vi "xijk_create_graphs_emission.vi"(7 "plot settings in":cluster{"axes in":T1, "plot colors in":T2} {"axes in"."precision of results" max=8 step=1}, 8 "error in":errorcluster, 11 "spectra in":T3) -> (0 "error out":errorcluster, 1 "Filter cube 2 emission":cluster{"Y":dbl[], "Y":dbl[]}[](graph), 3 "Filter cube 1 emission":cluster{"Y":dbl[], "Y":dbl[]}[](graph))   [LabVIEW 2010]
uses:
  Type Def/spectrum_table_control.ctl
  Type Def/axis_parameters.ctl
  revised version/Type Def/color_parameters.ctl
panel:
  # "Dichroic"
  # "Ex/Em filter"
  # "Fluorophore 1"
  # "Fluorophore 2"
  # "Laser /\nextra Em filter"
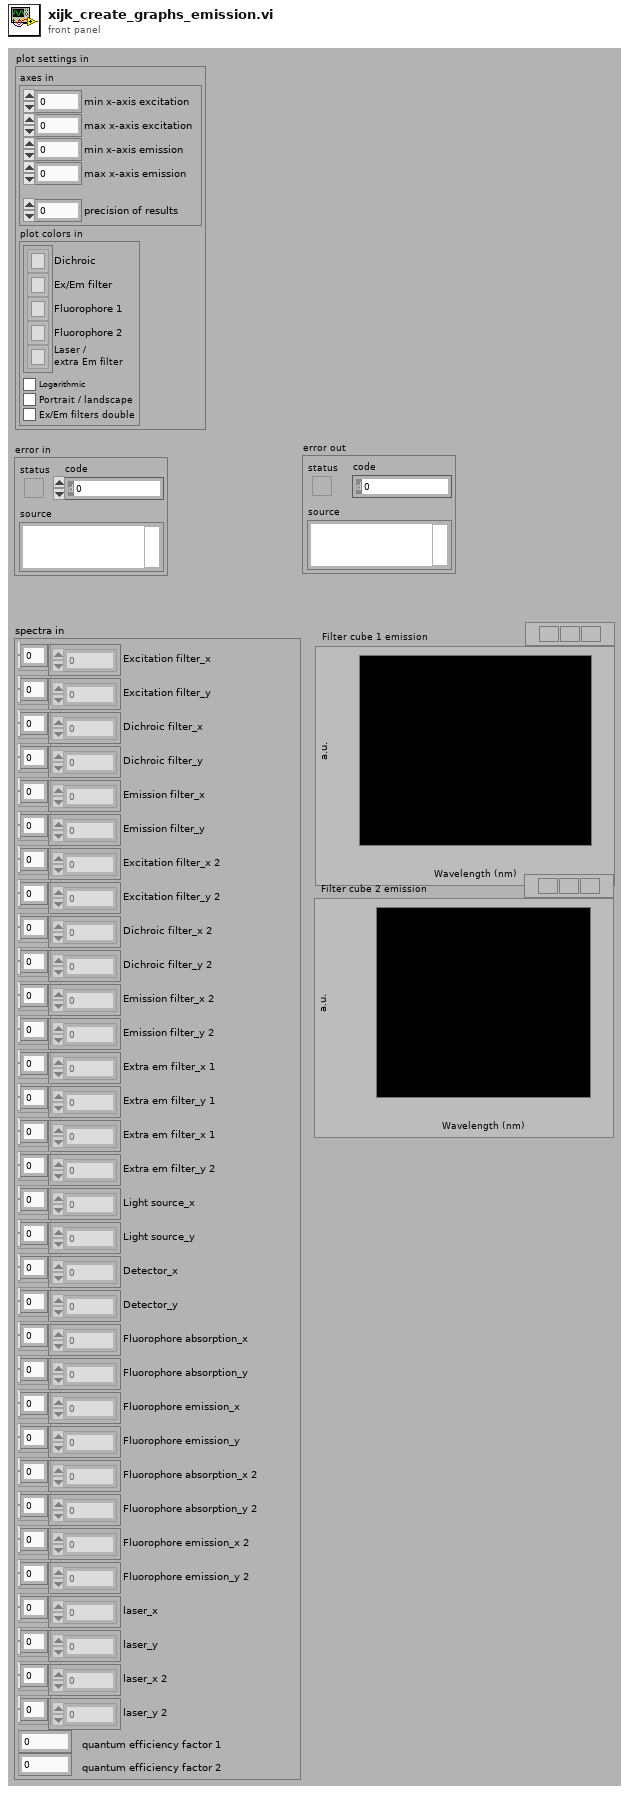
[diagram p1: front panel]
types:
  T1 = typedef "axis_parameters.ctl" = cluster{"min x-axis excitation":u16, "max x-axis excitation":u16, "min x-axis emission":u16, "max x-axis emission":u16, "precision of results":u8}
  T2 = typedef "color_parameters.ctl" = cluster{"Line colors":u32[], "Lanscape Portrait":bool, "Plot logarithmic":bool, "Ex/Em filters double":bool}
  T3 = typedef "spectrum_table_control.ctl" = cluster{"Excitation filter_x":i16[], "Excitation filter_y":dbl[], "Dichroic filter_x":i16[], "Dichroic filter_y":dbl[], "Emission filter_x":i16[], "Emission filter_y":dbl[], "Excitation filter_x 2":i16[], "Excitation filter_y 2":dbl[], "Dichroic filter_x 2":i16[], "Dichroic filter_y 2":dbl[], "Emission filter_x 2":i16[], "Emission filter_y 2":dbl[], "Extra em filter_x 1":i16[], "Extra em filter_y 1":dbl[], "Extra em filter_x 1":i16[], "Extra em filter_y 2":dbl[], "Light source_x":i16[], "Light source_y":dbl[], "Detector_x":i16[], "Detector_y":dbl[], "Fluorophore absorption_x":i16[], "Fluorophore absorption_y":dbl[], "Fluorophore emission_x":i16[], "Fluorophore emission_y":dbl[], "Fluorophore absorption_x 2":i16[], "Fluorophore absorption_y 2":dbl[], "Fluorophore emission_x 2":i16[], "Fluorophore emission_y 2":dbl[], "laser_x":i16[], "laser_y":dbl[], "laser_x 2":i16[], "laser_y 2":dbl[], "quantum efficiency factor 1":dbl, "quantum efficiency factor 2":dbl}
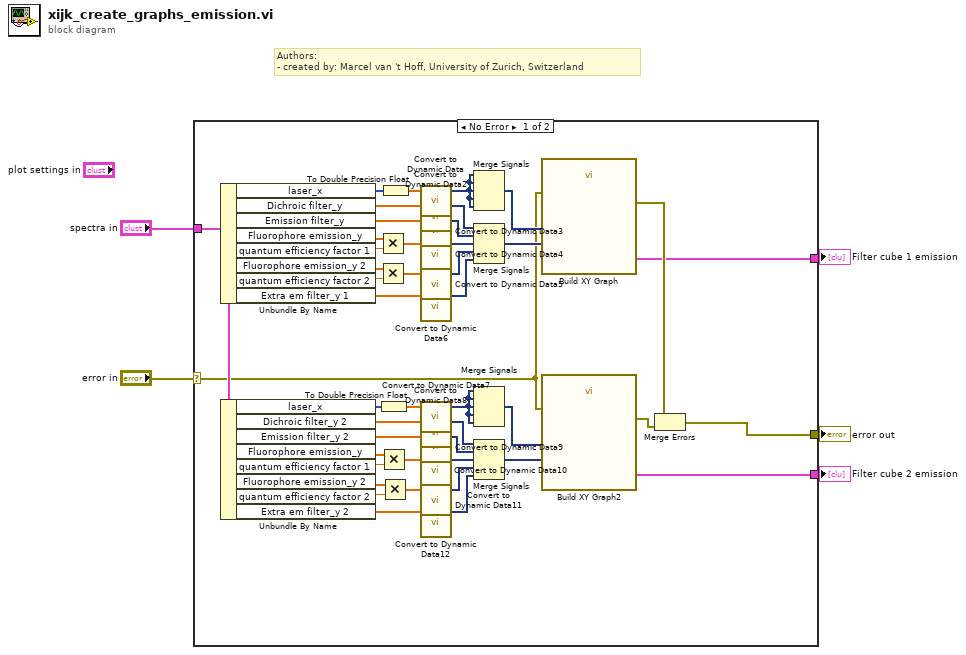
[diagram p0: block diagram]
diagram:
  # "Authors: \n- created by: Marcel van 't Hoff, University of Zurich, Switzerland"
  n1 = case shown="No Error" "error in" {
    selector: "error in" -> [w22 w51]
    tunnel: "spectra in" -> [w50 _]
    tunnel: [w23 w51] -> w4
    tunnel: [w6 _] -> w2
    tunnel: [w21 _] -> w1
    frame No Error {
      n2 = Unbundle By Name(w50) -> ("laser_x"=w49:i16[], "Dichroic filter_y"=w48:dbl[], "Emission filter_y"=w45:dbl[], "Fluorophore emission_y"=w43:dbl[], "quantum efficiency factor 1"=w16:dbl, "Fluorophore emission_y 2"=w18:dbl[], "quantum efficiency factor 2"=w14:dbl, "Extra em filter_y 1"=w40:dbl[])
      n3 = Unbundle By Name(w50) -> ("laser_x"=w29:i16[], "Dichroic filter_y 2"=w28:dbl[], "Emission filter_y 2"=w27:dbl[], "Fluorophore emission_y"=w8:dbl[], "quantum efficiency factor 1"=w12:dbl, "Fluorophore emission_y 2"=w10:dbl[], "quantum efficiency factor 2"=w11:dbl, "Extra em filter_y 2"=w26:dbl[])
      n4 = Multiply(x=w43, y=w16) -> (x*y=w17:dbl[])
      n5 = Multiply(x=w18, y=w14) -> (x*y=w15:dbl[])
      n6 = To Double Precision Float(number=w29) -> (double precision float=w20:dbl[])
      n7 = Multiply(x=w8, y=w12) -> (x*y=w7:dbl[])
      n8 = Multiply(x=w10, y=w11) -> (x*y=w9:dbl[])
      n9 = To Double Precision Float(number=w49) -> (double precision float=w19:dbl[])
      n10 = call "Convert to Dynamic Data"("Array"=w19) -> ("Dynamic Data Type"=w38:dynamicdata)  [unwired: 3 in]
      n11 = call "Convert to Dynamic Data2"("Array"=w48) -> ("Dynamic Data Type"=w47:dynamicdata)  [unwired: 3 in]
      n12 = call "Convert to Dynamic Data3"("Array"=w45) -> ("Dynamic Data Type"=w44:dynamicdata)  [unwired: 3 in]
      n13 = call "Convert to Dynamic Data4"("Array"=w17) -> ("Dynamic Data Type"=w42:dynamicdata)  [unwired: 3 in]
      n14 = call "Convert to Dynamic Data5"("Array"=w15) -> ("Dynamic Data Type"=w41:dynamicdata)  [unwired: 3 in]
      n15 = call "Convert to Dynamic Data6"("Array"=w40) -> ("Dynamic Data Type"=w39:dynamicdata)  [unwired: 3 in]
      n16 = call "Convert to Dynamic Data7"("Array"=w20) -> ("Dynamic Data Type"=w35:dynamicdata)  [unwired: 3 in]
      n17 = call "Convert to Dynamic Data8"("Array"=w28) -> ("Dynamic Data Type"=w30:dynamicdata)  [unwired: 3 in]
      n18 = call "Convert to Dynamic Data9"("Array"=w27) -> ("Dynamic Data Type"=w32:dynamicdata)  [unwired: 3 in]
      n19 = call "Convert to Dynamic Data10"("Array"=w7) -> ("Dynamic Data Type"=w33:dynamicdata)  [unwired: 3 in]
      n20 = call "Convert to Dynamic Data11"("Array"=w9) -> ("Dynamic Data Type"=w34:dynamicdata)  [unwired: 3 in]
      n21 = call "Convert to Dynamic Data12"("Array"=w26) -> ("Dynamic Data Type"=w13:dynamicdata)  [unwired: 3 in]
      n22 = Merge Signals(w38, w38, w38, w38, w38) -> (w37:dynamicdata)
      n23 = Merge Signals(w47, w44, w42, w41, w39) -> (w46:dynamicdata)
      n24 = Merge Signals(w35, w35, w35, w35, w35) -> (w36:dynamicdata)
      n25 = Merge Signals(w30, w32, w33, w34, w13) -> (w31:dynamicdata)
      n26 = call "Build XY Graph"("error in (no error)"=w22, "Y Input"=w46, "X Input"=w37) -> ("error out"=w25:errorcluster, "XY Graph"=w21:cluster{"Y":dbl[], "Y":dbl[]}[])  [unwired: 7 in]
      n27 = call "Build XY Graph2"("error in (no error)"=w22, "Y Input"=w31, "X Input"=w36) -> ("error out"=w24:errorcluster, "XY Graph"=w6:cluster{"Y":dbl[], "Y":dbl[]}[])  [unwired: 7 in]
      n28 = Merge Errors(w25, w24) -> (w23:errorcluster)
    }
    frame Error {
    }
  }
  "error out" <- w4
  "Filter cube 1 emission" <- w1
  "Filter cube 2 emission" <- w2
